vi "Check Error and Get Call Result.vi"(7 "AWS Core":refnum<class "HTTP Request.lvclass">, 8 "error in (no error)":errorcluster, 10 "Response body":string, 11 "Response header":string) -> (0 "error out":errorcluster, 1 "Redirect endpoint":string, 2 "500 Or Throttled?":bool=TRUE, 3 "Call Result":string)   [LabVIEW 2015, in "NI_AWS_Core.lvlib" / "HTTP Request.lvclass"]
doc: "Check the respnse header and body if necessary to obtain the call's result (Success or Error codes)."
uses:
  HTTP Request.lvclass
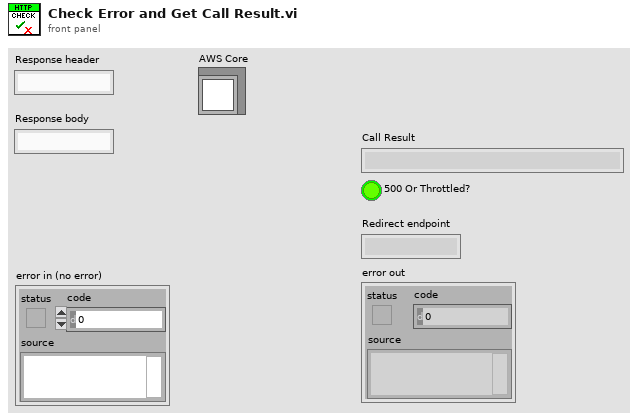
[diagram p1: front panel]
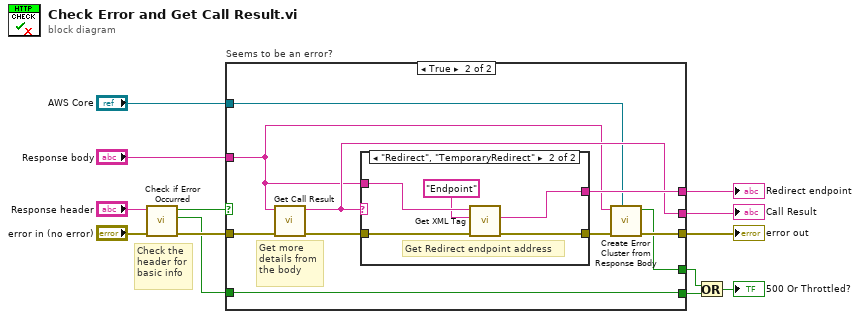
[diagram p0: block diagram]
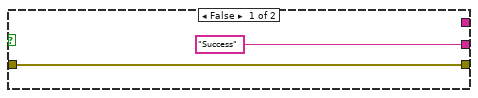
[diagram p2: hidden frame]
diagram:
  # "Check the\nheader for\nbasic info"
  n1 = call "Check if Error Occurred.vi"("error in (no error)"="error in (no error)", "Response header"="Response header") -> ("error out"=w10:errorcluster, "500 Error"=w5:bool, "Error Occurred"=w11:bool)  [unwired: 7 in]
  n2 = case "Seems to be an error?" shown="True" w11 {
    tunnel: w10 -> [w15 w25]
    tunnel: "Response body" -> [_ w19]
    tunnel: [w15 w20] -> w7
    tunnel: ["Success" ("Call Result") w23] -> w8
    tunnel: [_ w24] -> w6
    tunnel: [_ w18] -> w2
    tunnel: [_ w17] -> w4
    tunnel: w5 -> [_ w17]
    tunnel: "AWS Core" -> [_ w16]
    frame False {
    }
    frame True {
      # "Get more\ndetails from\nthe body"
      n3 = call "Get Call Result.vi"("error in (no error)"=w25, "Response body"=w19) -> ("error out"=w22:errorcluster, "Call Result"=w23:string)  [unwired: 8 in]
      n4 = case shown="\"Redirect\", \"TemporaryRedirect\"" w23 {
        tunnel: w19 -> [_ w31]
        tunnel: [_ w29] -> w24
        tunnel: [w26 w28] -> w21
        tunnel: w22 -> [w26 w27]
        frame Default {
        }
        frame "Redirect", "TemporaryRedirect" {
          # "Get Redirect endpoint address"
          n5 = call "Get XML Tag.vi"("error in (no error)"=w27, "Tag name"="Endpoint", "XML String in"=w31) -> ("error out"=w28:errorcluster, "Tag value"=w29:string)  [unwired: 4 in, 3 out]
        }
      }
      n6 = call "Create Error Cluster from Response Body.vi"("AWS Core"=w16, "error in (no error)"=w21, "Response body"=w19) -> ("error out"=w20:errorcluster, "Is Throttled?"=w18:bool)  [unwired: 7 in]
    }
  }
  "Call Result" <- w8
  "error out" <- w7
  "Redirect endpoint" <- w6
  n7 = Or(x=w2, y=w4) -> (x .or. y?=→"500 Or Throttled?":bool)
